vi "Siglent SPD3000 Series Timed Output.vi"() -> ()   [LabVIEW 2015]
doc: "This example shows how to configure the instrument's output to turn on with specified settings using the output timer.\n\n<B>Note:</B>\nThis example is invalid for the SPD3303C models."
uses:
  <instrlib>/Siglent SPD3000 Series/Siglent SPD3000 Series.lvlib
panel:
  in  "Enable Timer (Disable)":bool
  in  "Channel (1:CH1)":u16(ring)=1 items=["CH1"=1, "CH2"=2]
  in  "Duration (0 s)":dbl min=0.0 max=10000.0 step=1.0
  in  "Current (0 A)":dbl min=0.0 max=3.2 format="%.3f"
  in  "Voltage (0 V)":dbl min=0.0 max=32.0 format="%.3f"
  in  "Duration (0 s)":dbl min=0.0 max=10000.0 step=1.0
  in  "Current (0 A)":dbl min=0.0 max=3.2 format="%.3f"
  in  "Voltage (0 V)":dbl min=0.0 max=32.0 format="%.3f"
  in  "Duration (0 s)":dbl min=0.0 max=10000.0 step=1.0
  in  "Current (0 A)":dbl min=0.0 max=3.2 format="%.3f"
  in  "Voltage (0 V)":dbl min=0.0 max=32.0 format="%.3f"
  in  "Duration (0 s)":dbl min=0.0 max=10000.0 step=1.0
  in  "Current (0 A)":dbl min=0.0 max=3.2 format="%.3f"
  in  "Voltage (0 V)":dbl min=0.0 max=32.0 format="%.3f"
  in  "Duration (0 s)":dbl min=0.0 max=10000.0 step=1.0
  in  "Current (0 A)":dbl min=0.0 max=3.2 format="%.3f"
  in  "Voltage (0 V)":dbl min=0.0 max=32.0 format="%.3f"
  in  "VISA resource name":refnum<visa-resource-name>
  # "(c) 2016 SIGLENT TECHNOLOGIES CO., LTD.   ALL RIGHTS RESERVED."
  # "Timer Group 5"
  # "Timer Group 4"
  # "Timer Group 1"
  # "Timer Group 3"
  # "Timer Group 2"
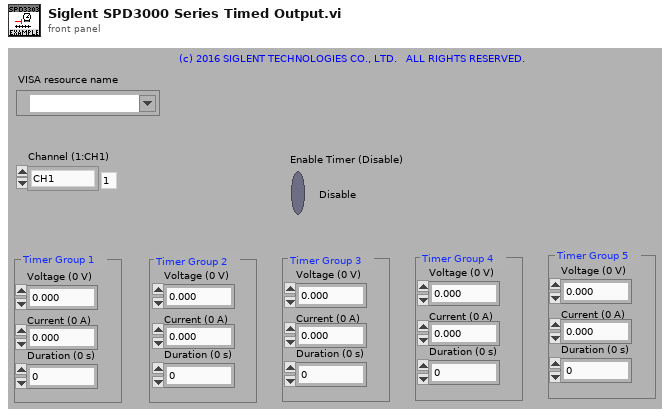
[diagram p1: front panel]
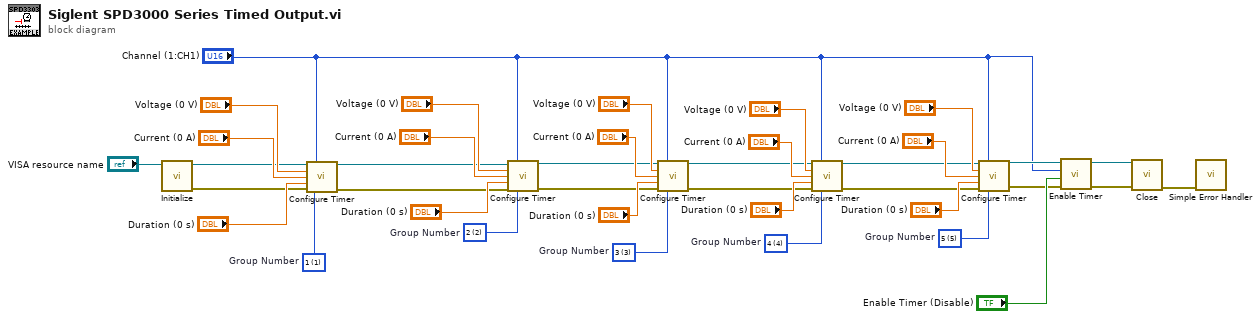
[diagram p0: block diagram]
diagram:
  w1 = u16 5 items=["1"=1, "2"=2, "3"=3, "4"=4, "5"=5]  # Group Number
  w2 = u16 4 items=["1"=1, "2"=2, "3"=3, "4"=4, "5"=5]  # Group Number
  w3 = u16 3 items=["1"=1, "2"=2, "3"=3, "4"=4, "5"=5]  # Group Number
  w4 = u16 2 items=["1"=1, "2"=2, "3"=3, "4"=4, "5"=5]  # Group Number
  w5 = u16 1 items=["1"=1, "2"=2, "3"=3, "4"=4, "5"=5]  # Group Number
  n1 = call <instrlib>:"Initialize.vi"("VISA resource name"="VISA resource name") -> ("error out"=w20:errorcluster, "VISA resource name out"=w21:refnum<visa-resource-name>)  [unwired: 9 in]
  n2 = call <instrlib>:"Configure Timer.vi"("VISA resource name"=w21, "Channel (1:CH1)"="Channel (1:CH1)", "Voltage (0 V)"="Voltage (0 V)", "Current (0 A)"="Current (0 A)", "Duration (0 s)"="Duration (0 s)", "error in (no error)"=w20, "Group Number (1:1)"=w5) -> ("VISA resource name out"=w19:refnum<visa-resource-name>, "error out"=w18:errorcluster)  [unwired: 7 in]
  n3 = call <instrlib>:"Configure Timer.vi"("VISA resource name"=w19, "Channel (1:CH1)"="Channel (1:CH1)", "Voltage (0 V)"="Voltage (0 V)", "Current (0 A)"="Current (0 A)", "Duration (0 s)"="Duration (0 s)", "error in (no error)"=w18, "Group Number (1:1)"=w4) -> ("VISA resource name out"=w17:refnum<visa-resource-name>, "error out"=w16:errorcluster)  [unwired: 7 in]
  n4 = call <instrlib>:"Configure Timer.vi"("VISA resource name"=w17, "Channel (1:CH1)"="Channel (1:CH1)", "Voltage (0 V)"="Voltage (0 V)", "Current (0 A)"="Current (0 A)", "Duration (0 s)"="Duration (0 s)", "error in (no error)"=w16, "Group Number (1:1)"=w3) -> ("VISA resource name out"=w15:refnum<visa-resource-name>, "error out"=w14:errorcluster)  [unwired: 7 in]
  n5 = call <instrlib>:"Configure Timer.vi"("VISA resource name"=w15, "Channel (1:CH1)"="Channel (1:CH1)", "Voltage (0 V)"="Voltage (0 V)", "Current (0 A)"="Current (0 A)", "Duration (0 s)"="Duration (0 s)", "error in (no error)"=w14, "Group Number (1:1)"=w2) -> ("VISA resource name out"=w13:refnum<visa-resource-name>, "error out"=w12:errorcluster)  [unwired: 7 in]
  n6 = call <instrlib>:"Configure Timer.vi"("VISA resource name"=w13, "Channel (1:CH1)"="Channel (1:CH1)", "Voltage (0 V)"="Voltage (0 V)", "Current (0 A)"="Current (0 A)", "Duration (0 s)"="Duration (0 s)", "error in (no error)"=w12, "Group Number (1:1)"=w1) -> ("VISA resource name out"=w10:refnum<visa-resource-name>, "error out"=w9:errorcluster)  [unwired: 7 in]
  n7 = call <instrlib>:"Enable Timer.vi"("error in (no error)"=w9, "Enable Timer (Disable)"="Enable Timer (Disable)", "Channel (1:CH1)"="Channel (1:CH1)", "VISA resource name"=w10) -> ("error out"=w6:errorcluster, "VISA resource name out"=w7:refnum<visa-resource-name>)  [unwired: 6 in]
  n8 = call <instrlib>:"Close.vi"("error in (no error)"=w6, "VISA resource name"=w7) -> ("error out"=w37:errorcluster)  [unwired: 9 in]
  n9 = call <vilib>:"Simple Error Handler.vi"("error in (no error)"=w37) -> ()  [unwired: 4 in, 5 out]
